vi "SynapseAPI-Set Tank (create).vi"(0 "URL":string="http://localhost:24414", 7 "tank":string, 11 "error in (no error)":errorcluster) -> (15 "error out":errorcluster)   [LabVIEW 2020]
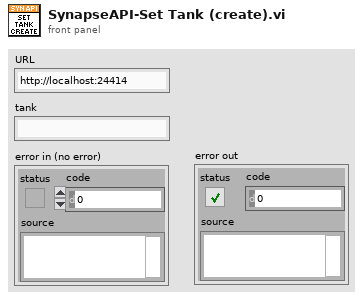
[diagram p1: front panel]
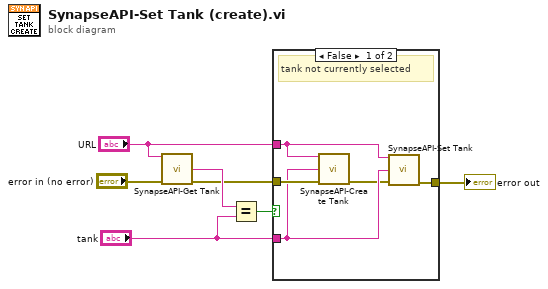
[diagram p0: block diagram]
diagram:
  n1 = call "SynapseAPI-Get Tank.vi"("URL"="URL", "error in (no error)"="error in (no error)") -> ("tank"=w6:string, "error out"=w4:errorcluster)  [unwired: 12 in]
  n2 = Equal?(x=w6, y="tank") -> (x = y?=w5:bool)
  n3 = case shown="False" w5 {
    tunnel: w4 -> [w11 w13]
    tunnel: "URL" -> [w12 _]
    tunnel: "tank" -> [w9 _]
    tunnel: [w10 w13] -> w1
    frame False {
      # "tank not currently selected"
      n4 = call "SynapseAPI-Create Tank.vi"("URL"=w12, "tank"=w9, "error in (no error)"=w11) -> ("error out"=w8:errorcluster)  [unwired: 12 in]
      n5 = call "SynapseAPI-Set Tank.vi"("URL"=w12, "tank"=w9, "error in (no error)"=w8) -> ("error out"=w10:errorcluster)  [unwired: 12 in]
    }
    frame True {
      # "tank already selected"
    }
  }
  "error out" <- w1
